vi "Rinocloud_HTTP_create_empty.vi"(4 "Extra metadata array":T2(array[cluster])=[{"Attribute"="", "Value"="", "Data type"=enum."<null>"}], 5 "Parent ID":string="name", 6 "error in (no error)":errorcluster, 7 "Notes":string, 8 "Tags":string, 9 "Name":string) -> (0 "error out":errorcluster, 3 "Status":T1={"headers"="", "body"="", "ID"="", "Saved"=TRUE})   [LabVIEW 2011, in "Rinocloud Library.lvlib"]
uses:
  Rinocloud Library.lvlib
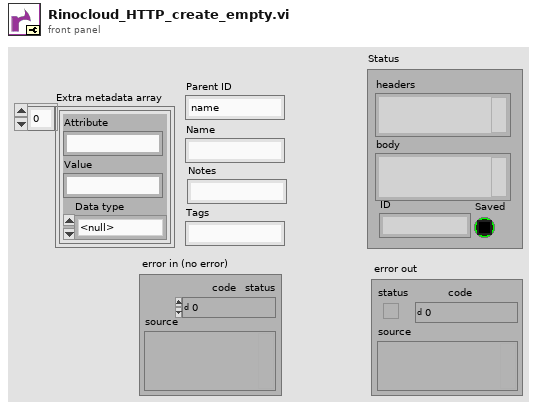
[diagram p1: front panel]
types:
  T1 = cluster{"headers":string, "body":string, "ID":string, "Saved":bool}
  T2 = cluster{"Attribute":string, "Value":string, "Data type":enum16{"Numeric", "String", "1D array of strings", "1D array of doubles", "Data JSON string", "<null>"}}[]
  T3 = cluster{"Name":string, "Notes":string, "Tags":string}
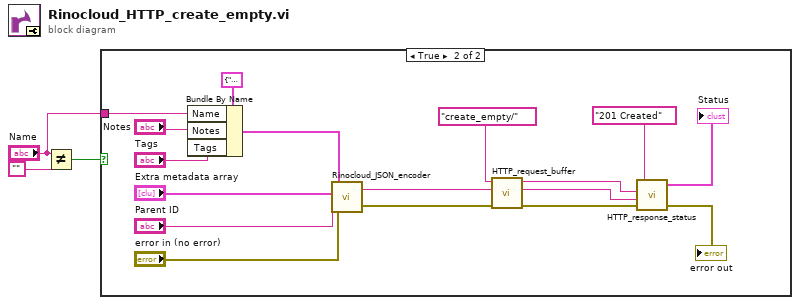
[diagram p0: block diagram]
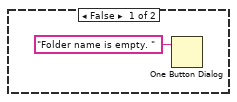
[diagram p2: hidden frame]
diagram:
  n1 = Not Equal?(x="Name", y="") -> (x != y?=w2:bool)
  n2 = case shown="True" w2 {
    tunnel: "Name" -> [_ w7]
    frame False {
      n3 = One Button Dialog(message="Folder name is empty. ") -> ()  [unwired: 1 in, 1 out]
    }
    frame True {
      n4 = Bundle By Name(cluster=T3 {"Name"="", "Notes"="", "Tags"=""} ("Metadata"), "Name"=w7, "Notes"="Notes", "Tags"="Tags") -> (w10:T3)
      n5 = call "Rinocloud_JSON_encoder.vi"("Metadata"=w10, "Extra metadata array"="Extra metadata array", "parent ID"="Parent ID", "error in (no error)"="error in (no error)") -> ("JSON payload"=w15:string, "error out"=w18:errorcluster)  [unwired: 1 in]
      n6 = call "HTTP_request_buffer.vi"("error in (no error)"=w18, "JSON payload"=w15, "Endpoint"="create_empty/") -> ("error out"=w19:errorcluster, "body"=w17:string, "headers"=w16:string)  [unwired: 2 in]
      n7 = call "HTTP_response_status.vi"("error in (no error)"=w19, "body"=w17, "headers"=w16, "HTTP status"="201 Created") -> ("error out"=→"error out":errorcluster, "Status"=→"Status":T1)  [unwired: 1 in]
    }
  }
